vi "Get Sensor.vi"(8 "error in (no error)":errorcluster, 10 "Name":string, 11 "Sensor List Class in":refnum<class "Sensor List Class.lvclass">) -> (0 "error out":errorcluster, 2 "Sensor DAO Out":refnum<class "Sensor DAO Class.lvclass">, 3 "Sensor List Class out":refnum<class "Sensor List Class.lvclass">)   [LabVIEW 2013, in "Sensor List Class.lvclass"]
uses:
  Sensor List Class.lvclass
  Sensor DAO Class.lvclass
  Sensor List Class.lvclass/Sensor List Class.ctl
panel:
  out "Metadata":string[](array[string])
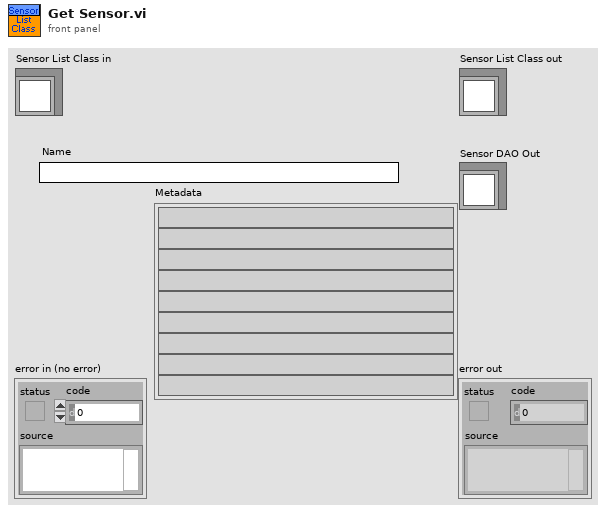
[diagram p1: front panel]
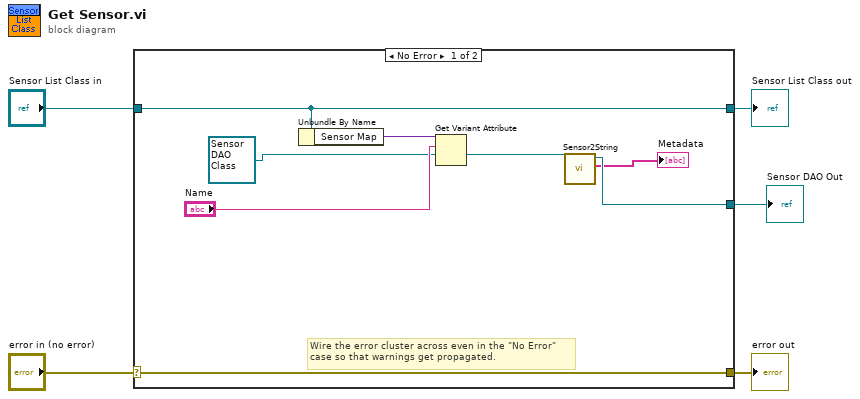
[diagram p0: block diagram]
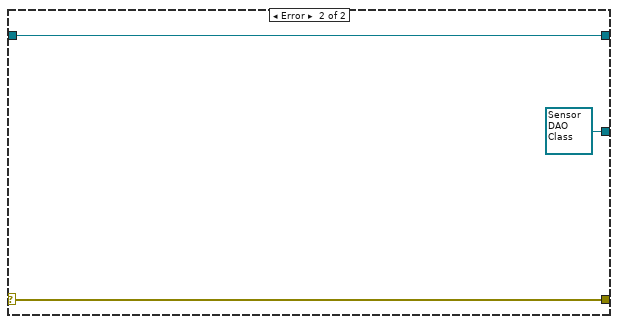
[diagram p2: hidden frame]
diagram:
  n1 = case shown="No Error" "error in (no error)" {
    selector: "error in (no error)" -> [w13 w16]
    tunnel: [w13 w16] -> w4
    tunnel: [w12 w15] -> w2
    tunnel: "Sensor List Class in" -> [w12 w15]
    tunnel: [w7 refnum<class "Sensor DAO Class.lvclass"> refnum ("Sensor DAO Out")] -> w1
    frame No Error {
      # "Wire the error cluster across even in the \"No Error\"\ncase so that warnings get propagated."
      n2 = Unbundle By Name(w12) -> ("Sensor Map"=w11:variant)
      n3 = Get Variant Attribute(Variant=w11, name="Name", default value (empty Variant)=refnum<class "Sensor DAO Class.lvclass"> refnum ("Sensor DAO Out")) -> (value=w8:refnum<class "Sensor DAO Class.lvclass">)  [unwired: 1 in, 3 out]
      n4 = call "Sensor2String.vi"("Sensor DAO Class in"=w8) -> ("Strings"=→"Metadata":string[], "Sensor DAO Class out"=w7:refnum<class "Sensor DAO Class.lvclass">)  [unwired: 8 in, 1 out]
    }
    frame Error {
    }
  }
  "error out" <- w4
  "Sensor List Class out" <- w2
  "Sensor DAO Out" <- w1
